vi "Test.vi"() -> ()   [LabVIEW 2019]
uses:
  CD Parameter Manager Class/CD Parameter Manager.lvclass
  Controls and Globals/Parameters.vi
panel:
  in  "stop":bool
  in  "Age":i32
  in  "Foreign?":bool
  in  "Height":dbl
  in  "Save to File":bool
  in  "Load from File":bool
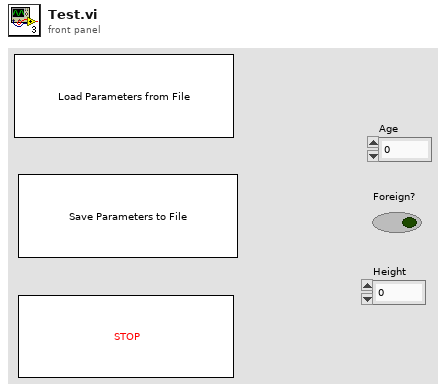
[diagram p1: front panel]
types:
  T1 = cluster{"Label":string, "Data type":enum16{"Double", "I32", "Boolean", "String"}}[]
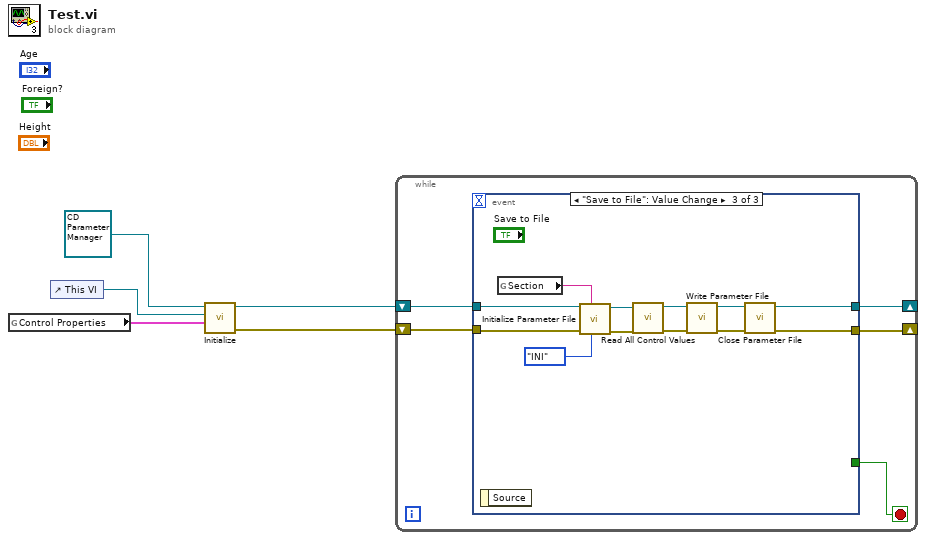
[diagram p0: block diagram]
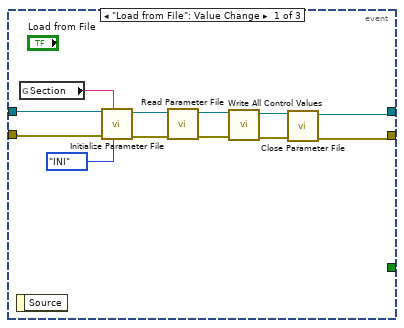
[diagram p2: hidden frame]
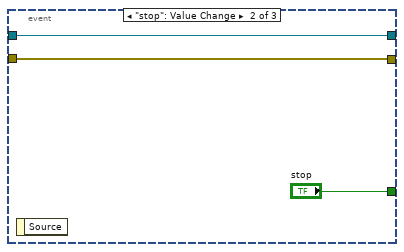
[diagram p3: hidden frame]
diagram:
  n1 = global read "Parameters.vi" "Control Properties"() -> (w5:T1)
  n2 = control-ref of="This VI"() -> (w4:refnum<vi>)
  n3 = call "Initialize.vi"("Control Properties"=w5, "VI Refnum"=w4, "CD Parameter Manager in"=refnum<class "CD Parameter Manager.lvclass"> refnum) -> ("error out"=w3:errorcluster, "CD Parameter Manager out"=w2:refnum<class "CD Parameter Manager.lvclass">)  [unwired: 7 in]
  n4 = while {
    shift-right: [w7] -> _
    shift-left: w2 -> [w9]
    shift-right: [w8] -> _
    shift-left: w3 -> [w10]
    stop <- w6 stop-if-true
    n5 = event shown="[2] \"Save to File\": Value Change" {
      selector: _ -> [_ _ _]
      dyn-events: _ -> [_ _ _]
      timeout: _ -> [_ _ _]
      tunnel: w10 -> [w13 w24 w35]
      tunnel: w9 -> [w14 w25 w34]
      tunnel: [w17 w24 w26] -> w8
      tunnel: [w18 w25 w28] -> w7
      tunnel: [_ "stop" _] -> w6
      event "Load from File": Value Change {
        n6 = event-data() -> ()  [unwired: 1 in, 1 out]
        n7 = global read "Parameters.vi" "Section"() -> (w16:string)
        n8 = call "Initialize Parameter File.vi"("File type"=enum16{"INI"}."INI", "Section"=w16, "error in (no error)"=w13, "CD Parameter Manager in"=w14) -> ("error out"=w12:errorcluster, "CD Parameter Manager out"=w11:refnum<class "CD Parameter Manager.lvclass">)  [unwired: 6 in]
        n9 = call "Read Parameter File.vi"("error in (no error)"=w12, "CD Parameter Manager in"=w11) -> ("error out"=w21:errorcluster, "CD Parameter Manager out"=w22:refnum<class "CD Parameter Manager.lvclass">)  [unwired: 8 in]
        n10 = call "Write All Control Values.vi"("error in (no error)"=w21, "CD Parameter Manager in"=w22) -> ("error out"=w19:errorcluster, "CD Parameter Manager out"=w20:refnum<class "CD Parameter Manager.lvclass">)  [unwired: 8 in]
        n11 = call "Close Parameter File.vi"("error in (no error)"=w19, "CD Parameter Manager in"=w20) -> ("error out"=w17:errorcluster, "CD Parameter Manager out"=w18:refnum<class "CD Parameter Manager.lvclass">)  [unwired: 8 in]
      }
      event "stop": Value Change {
        n12 = event-data() -> ()  [unwired: 1 in, 1 out]
      }
      event "Save to File": Value Change {
        n13 = event-data() -> ()  [unwired: 1 in, 1 out]
        n14 = global read "Parameters.vi" "Section"() -> (w37:string)
        n15 = call "Initialize Parameter File.vi"("File type"=enum16{"INI"}."INI", "Section"=w37, "error in (no error)"=w35, "CD Parameter Manager in"=w34) -> ("error out"=w32:errorcluster, "CD Parameter Manager out"=w33:refnum<class "CD Parameter Manager.lvclass">)  [unwired: 6 in]
        n16 = call "Read All Control Values.vi"("error in (no error)"=w32, "CD Parameter Manager in"=w33) -> ("error out"=w31:errorcluster, "CD Parameter Manager out"=w30:refnum<class "CD Parameter Manager.lvclass">)  [unwired: 8 in]
        n17 = call "Write Parameter File.vi"("error in (no error)"=w31, "CD Parameter Manager in"=w30) -> ("error out"=w27:errorcluster, "CD Parameter Manager out"=w29:refnum<class "CD Parameter Manager.lvclass">)  [unwired: 8 in]
        n18 = call "Close Parameter File.vi"("error in (no error)"=w27, "CD Parameter Manager in"=w29) -> ("error out"=w26:errorcluster, "CD Parameter Manager out"=w28:refnum<class "CD Parameter Manager.lvclass">)  [unwired: 8 in]
      }
    }
  }
